vi "set_plane_or_volume_repetitions.vi"(8 "error in (no error)":errorcluster, 10 "repetitions per frame":i32, 11 "TrajectoryAK101022Resonance in":refnum<class "TrajectoryAK101022Resonance.lvclass">) -> (0 "error out":errorcluster, 3 "TrajectoryAK101022Resonance out":refnum<class "TrajectoryAK101022Resonance.lvclass">)   [LabVIEW 2010, in "TrajectoryAK101022Resonance.lvclass"]
uses:
  TrajectoryAK101022Resonance.lvclass
  TrajectoryAK101022Resonance.lvclass/TrajectoryAK101022Resonance.ctl
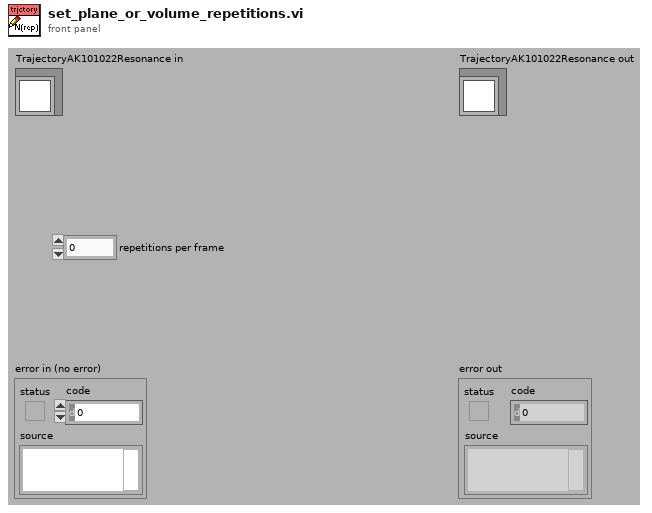
[diagram p1: front panel]
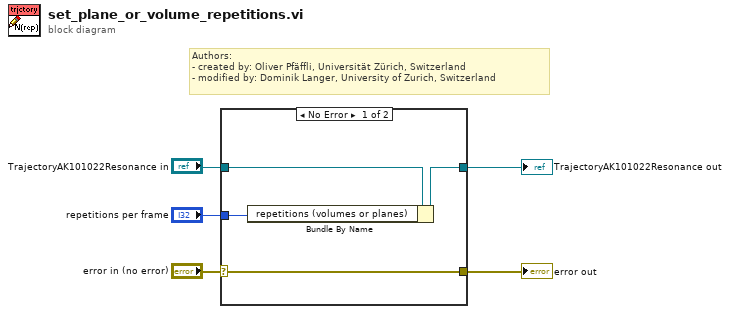
[diagram p0: block diagram]
diagram:
  # "Authors: \n- created by: Oliver Pfäffli, Universität Zürich, Switzerland\n- modified by: Dominik Langer, University of Zurich, Switzerland"
  n1 = case shown="No Error" "error in (no error)" {
    selector: "error in (no error)" -> [w9 w11]
    tunnel: [w9 w11] -> w5
    tunnel: [w7 w10] -> w4
    tunnel: "TrajectoryAK101022Resonance in" -> [w8 w10]
    tunnel: "repetitions per frame" -> [w6 _]
    frame No Error {
      n2 = Bundle By Name(cluster=w8, "repetitions (volumes or planes)"=w6) -> (w7:refnum<class "TrajectoryAK101022Resonance.lvclass">)
    }
    frame Error {
    }
  }
  "error out" <- w5
  "TrajectoryAK101022Resonance out" <- w4
